vi "Parse Command.vi"(11 "text":string) -> (1 "Commands":string[](array[string]), 2 "flute dia (in)":dbl, 3 "cmd amd State":cluster{"Command":string, "End State":dbl[]}[](array[cluster]))   [LabVIEW 2024]
uses:
  <vilib>/Utility/error.llb/Trim Whitespace One-Sided.vi
panel:
  out "inch?":bool
  out "header":string[](array[string])
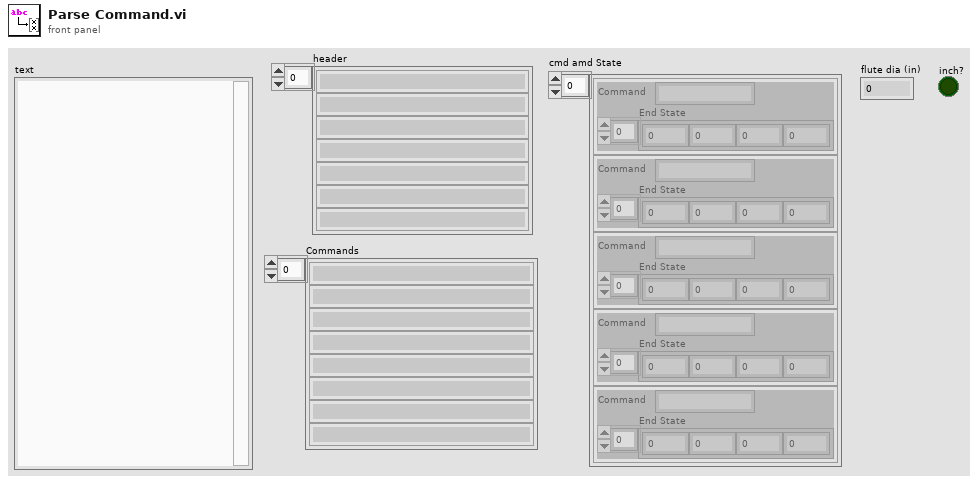
[diagram p1: front panel]
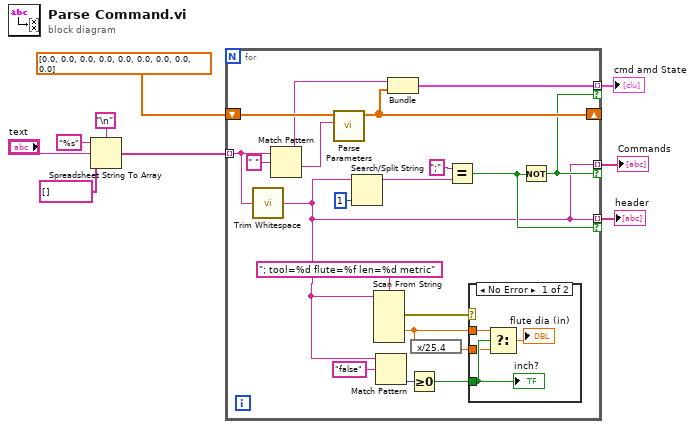
[diagram p0: block diagram]
diagram:
  n1 = Spreadsheet String To Array(delimiter (Tab)="\n", format string="%s", spreadsheet string="text", array type (2D Dbl)=string[] [] ("appended array")) -> (array=w3:string[])
  n2 = for {
    tunnel: w3 -> [w23] mode=indexing
    shift-right: [w25] -> _
    shift-left: dbl[] [0.0, 0.0, 0.0, 0.0, 0.0, 0.0, 0.0, 0.0, 0.0] -> [w27]
    tunnel: [w24] -> w5 mode=indexing if=w13
    tunnel: [w10] -> w4 mode=indexing if=w20
    tunnel: [w10] -> w2 mode=indexing if=w13
    n3 = call <vilib>:"Trim Whitespace.vi"("string"=w23) -> ("trimmed string"=w10:string)  [unwired: 1 in]
    n4 = Match Pattern(string=w23, regular expression=" ") -> (before substring=w26:string, after substring=w28:string)  [unwired: 1 in, 2 out]
    n5 = call <userlib>:"Parse Parameters.vi"("String"=w28, "Array in"=w27) -> ("Array out"=w25:dbl[])  [unwired: 9 in]
    n6 = Search/Split String(string=w10, offset (0)=1) -> (substring before match=w12:string)  [unwired: 1 in, 2 out]
    n7 = Scan From String(format string="; tool=%d flute=%f len=%d metric" ("regular expression"), input string=w10) -> (error out=w18:errorcluster, output 2=w11:dbl)  [unwired: 7 in, 2 out]
    n8 = Match Pattern(string=w10, regular expression="false") -> (offset past match=w16:i32)  [unwired: 1 in, 3 out]
    n9 = Bundle("text"=w26, "Array out"=w25) -> (w24:cluster{"text":string, "Array out":dbl[]})  [unwired: 1 in]
    n10 = Greater Or Equal To 0?(x=w16) -> (x >= 0?=w15:bool)
    n11 = expression code="x/25.4"(w11) -> (w14:dbl)
    n12 = Equal?(x=";", y=w12) -> (x = y?=w20:bool)
    n13 = case shown="No Error" w18 {
      tunnel: w11 -> [w33 _]
      tunnel: w15 -> [w32 _]
      tunnel: w14 -> [w30 _]
      frame No Error {
        n14 = Select(t=w33, s=w32, f=w30) -> (s? t:f=→"flute dia (in)":dbl)
        "inch?" <- w32
      }
      frame Error {
      }
    }
    n15 = Not(x=w20) -> (.not. x?=w13:bool)
  }
  "Commands" <- w2
  "cmd amd State" <- w5
  "header" <- w4
